vi "Create System Channels.vi"(8 "error in (no error)":errorcluster, 11 "Parent Ref in":T4 format="%.0x") -> (0 "error out":errorcluster, 3 "Parent Ref out":T4 format="%.0x")   [LabVIEW 2016, in "DCM System Explorer.lvlib"]
uses:
  DCM System Explorer.lvlib
  <vilib>/NI Veristand/Custom Device API/Custom Device Item Ref.ctl
  <vilib>/Powertrain Controls/Device Drivers/DCM/Rev0/RT/System State.ctl
  <vilib>/Powertrain Controls/Device Drivers/DCM/Rev0/RT/System ADC.ctl
  <vilib>/Powertrain Controls/Device Drivers/DCM/Rev0/RT/Internal Fault.ctl
  <vilib>/NI Veristand/Custom Device API/Custom Device Channel Type.ctl
  Shared/DCM Constants and GUIDs.vi
  Shared/DCM Properties.vi
  <vilib>/NI VeriStand/Custom Device API/Custom Device API.lvlib
  DCM Shared.lvlib
  <vilib>/Powertrain Controls/Device Drivers/DCM/Rev0/RT/DCM - RT.lvclass
panel:
  out "Status":T1 {"System ADC"."Fan [V]" format="%#_3p"; "System ADC"."Primary B1B2 [V]" format="%#_3p"; "System ADC"."Primary B3B4 [V]" format="%#_3p"; "System ADC"."Primary A3A4 [V]" format="%#_3p"; "System ADC"."Primary A1A2 [V]" format="%#_3p"; "System ADC"."MPRD [V]" format="%#_3p"; "System ADC"."Ext HV B [V]" format="%#_3p"; "System ADC"."Ext HV A [V]" format="%#_3p"; "System ADC"."Pump Zener B [V]" format="%#_3p"; "System ADC"."Pump Zener A [V]" format="%#_3p"; "System ADC"."DI Zener B [V]" format="%#_3p"; "System ADC"."DI Zener A [V]" format="%#_3p"; "System ADC"."Key [V]" format="%#_3p"; "System ADC"."DRVP [V]" format="%#_3p"; "System ADC"."Battery [V]" format="%#_3p"; "System ADC"."FET Driver [V]" format="%#_3p"; "System ADC"."Secondary B1B2 [V]" format="%#_3p"; "System ADC"."Secondary B3B4 [V]" format="%#_3p"; "System ADC"."Secondary A3A4 [V]" format="%#_3p"; "System ADC"."Secondary A1A2 [V]" format="%#_3p"; "System ADC"."Primary Range [V]" format="%#_3p"; "System ADC"."Temp Boost B [C]" format="%#_3p"; "System ADC"."Temp Primary A [C]" format="%#_3p"; "System ADC"."Temp Secondary A [C]" format="%#_3p"; "System ADC"."Temp Fan Intake [C]" format="%#_3p"; "System ADC"."Temp CPU [C]" format="%#_3p"; "System ADC"."Temp DI Zener B [C]" format="%#_3p"; "System ADC"."Temp DI B [C]" format="%#_3p"; "System ADC"."Temp DI Zener A [C]" format="%#_3p"; "System ADC"."Temp DI A [C]" format="%#_3p"; "System ADC"."Temp HH 7-12 [C]" format="%#_3p"; "System ADC"."Temp HH 1-6 [C]" format="%#_3p"; "System ADC"."AI 12 [V]" format="%#_3p"; "System ADC"."AI 11 [V]" format="%#_3p"; "System ADC"."AI 10 [V]" format="%#_3p"; "System ADC"."AI 9 [V]" format="%#_3p"; "System ADC"."AI 8 [V]" format="%#_3p"; "System ADC"."AI 7 [V]" format="%#_3p"; "System ADC"."AI 6 [V]" format="%#_3p"; "System ADC"."AI 5 [V]" format="%#_3p"; "System ADC"."AI 4 [V]" format="%#_3p"; "System ADC"."AI 3 [V]" format="%#_3p"; "System ADC"."AI 2 [V]" format="%#_3p"; "System ADC"."AI 1 [V]" format="%#_3p"}
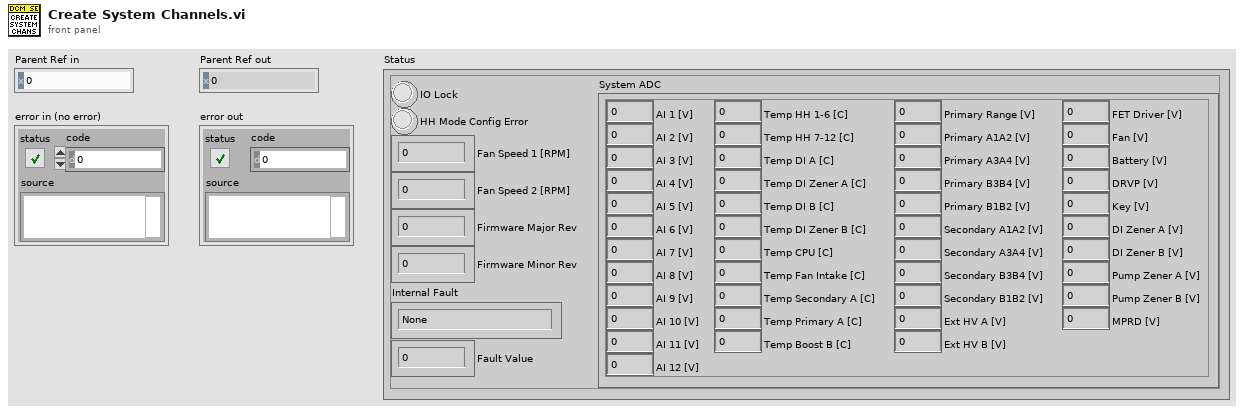
[diagram p1: front panel]
types:
  T1 = typedef "DCM - RT.lvclass/System State.ctl" = cluster{"System ADC":T2, "IO Lock":bool, "HH Mode Config Error":bool, "Fan Speed 1 [RPM]":sgl, "Fan Speed 2 [RPM]":sgl, "Firmware Major Rev":u16, "Firmware Minor Rev":u16, "Internal Fault":T3, "Fault Value":dbl}
  T2 = typedef "DCM - RT.lvclass/System ADC.ctl" = cluster{"AI 1 [V]":sgl, "AI 2 [V]":sgl, "AI 3 [V]":sgl, "AI 4 [V]":sgl, "AI 5 [V]":sgl, "AI 6 [V]":sgl, "AI 7 [V]":sgl, "AI 8 [V]":sgl, "AI 9 [V]":sgl, "AI 10 [V]":sgl, "AI 11 [V]":sgl, "AI 12 [V]":sgl, "Temp HH 1-6 [C]":sgl, "Temp HH 7-12 [C]":sgl, "Temp DI A [C]":sgl, "Temp DI Zener A [C]":sgl, "Temp DI B [C]":sgl, "Temp DI Zener B [C]":sgl, "Temp CPU [C]":sgl, "Temp Fan Intake [C]":sgl, "Temp Secondary A [C]":sgl, "Temp Primary A [C]":sgl, "Temp Boost B [C]":sgl, "Primary Range [V]":sgl, "Primary A1A2 [V]":sgl, "Primary A3A4 [V]":sgl, "Primary B3B4 [V]":sgl, "Primary B1B2 [V]":sgl, "Secondary A1A2 [V]":sgl, "Secondary A3A4 [V]":sgl, "Secondary B3B4 [V]":sgl, "Secondary B1B2 [V]":sgl, "Ext HV A [V]":sgl, "Ext HV B [V]":sgl, "FET Driver [V]":sgl, "Fan [V]":sgl, "Battery [V]":sgl, "DRVP [V]":sgl, "Key [V]":sgl, "DI Zener A [V]":sgl, "DI Zener B [V]":sgl, "Pump Zener A [V]":sgl, "Pump Zener B [V]":sgl, "MPRD [V]":sgl}
  T3 = typedef "DCM - RT.lvclass/Internal Fault.ctl" = enum32{"None", "Temp HH 1-6", "Temp HH 7-12", "Temp DI A", "Temp DI Zener A", "Temp DI B", "Temp DI Zener B", "Temp Intake", "Temp Primary A", "Temp Secondary A", "Temp Boost B", "Temp CPU", "Low Battery", "Inrush Protection", "A Run Enable", "B Run Enable"}
  T4 = typedef "Custom Device API.lvlib/Custom Device Item Ref.ctl" = u64
  T5 = typedef "Custom Device API.lvlib/Custom Device Channel Type.ctl" = enum16{"Input", "Output"}
  T6 = typedef "DCM Shared.lvlib/Channel.ctl" = cluster{"Name":string, "Units":string, "Default":dbl, "Description":string}
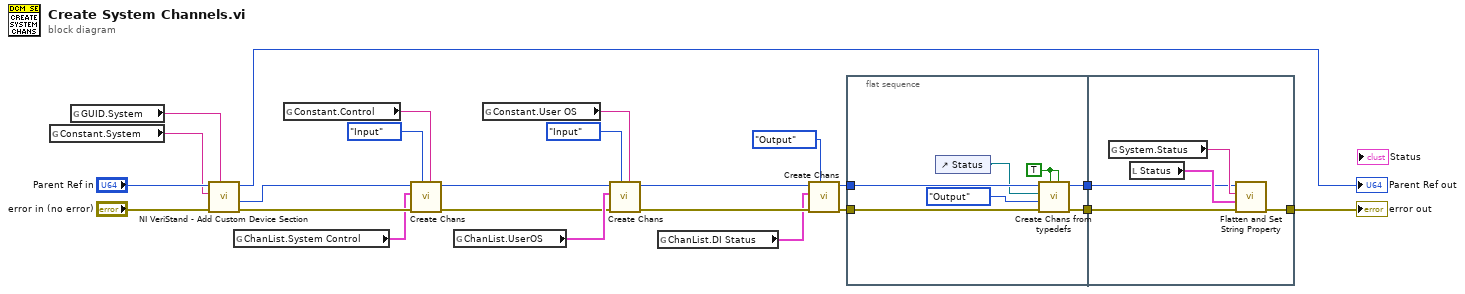
[diagram p0: block diagram]
diagram:
  n1 = global read "DCM Constants and GUIDs.vi" "Constant.System"() -> (w22:string)
  n2 = global read "DCM Constants and GUIDs.vi" "GUID.System"() -> (w21:string)
  n3 = call <vilib>:"NI VeriStand - Add Custom Device Section.vi"("GUID (Default Section)"=w21, "error in (no error)"="error in (no error)", "Section Name"=w22, "Parent Ref in"="Parent Ref in") -> ("error out"=w17:errorcluster, "Section Ptr"=w19:T4, "Parent Ref out"=→"Parent Ref out":T4)  [unwired: 4 in, 1 out]
  n4 = global read "DCM Constants and GUIDs.vi" "ChanList.System Control"() -> (w16:T6[])
  n5 = global read "DCM Constants and GUIDs.vi" "Constant.Control"() -> (w18:string)
  n6 = call "Create Chans.vi"("New Section Name (none)"=w18, "Type"=Custom_Device_Channel_Type."Input", "error in (no error)"=w17, "Channels"=w16, "Section Ptr"=w19) -> ("error out"=w7:errorcluster, "Section Ptr dup"=w8:T4)  [unwired: 3 in, 2 out]
  n7 = global read "DCM Constants and GUIDs.vi" "ChanList.UserOS"() -> (w9:T6[])
  n8 = global read "DCM Constants and GUIDs.vi" "Constant.User OS"() -> (w10:string)
  n9 = call "Create Chans.vi"("New Section Name (none)"=w10, "Type"=Custom_Device_Channel_Type."Input", "error in (no error)"=w7, "Channels"=w9, "Section Ptr"=w8) -> ("error out"=w5:errorcluster, "Section Ptr dup"=w6:T4)  [unwired: 3 in, 2 out]
  n10 = global read "DCM Constants and GUIDs.vi" "ChanList.DI Status"() -> (w2:T6[])
  n11 = call "Create Chans.vi"("Type"=Custom_Device_Channel_Type."Output", "error in (no error)"=w5, "Channels"=w2, "Section Ptr"=w6) -> ("error out"=w3:errorcluster, "Section Ptr dup"=w4:T4)  [unwired: 4 in, 2 out]
  n12 = flat-sequence {
    tunnel: [w29] -> w14
    tunnel: [w28] -> w13
    tunnel: w4 -> [w27]
    tunnel: w3 -> [w26]
    tunnel: [w34] -> w12
    tunnel: w14 -> [w32]
    tunnel: w13 -> [w36]
    frame #0 {
      w31 = TRUE ("Prevent overwrite? (F)")
      n13 = control-ref of="Status"() -> (w25:refnum<vi>)
      n14 = call "Create Chans from typedefs.vi"("Default from text? (F)"=w31, "Prevent overwrite? (F)"=w31, "error in"=w26, "Type"=Custom_Device_Channel_Type."Output", "Ctl Ref"=w25, "Section Ref in"=w27) -> ("error out"=w28:errorcluster, "Section Ref out"=w29:T4)  [unwired: 3 in, 1 out]
    }
    frame #1 {
      n15 = global read "DCM Properties.vi" "System.Status"() -> (w35:string)
      n16 = local read "Status"() -> (w33:T1)
      n17 = call "Flatten and Set String Property.vi"("error in (no error)"=w36, "Value"=w33, "Property Name"=w35, "Section Ref in"=w32) -> ("error out"=w34:errorcluster)  [unwired: 6 in, 1 out]
    }
  }
  "error out" <- w12
